vi "test_COM_comando1byte.vi"() -> ()   [LabVIEW 2019]
uses:
  <vilib>/numeric/Random Number (Range) U64.vi
  <vilib>/numeric/sub_Random U32.vi
  <vilib>/Instr/_visa.llb/VISA Configure Serial Port (Instr).vi
panel:
  out "x = y?":bool
  out "bytes enviados":u32
  out "error out":errorcluster
  out "numero de tramas\ncorrectamente recibidas":i64
  out "cmd enviado":string
  out "cmd leido":string
  in  "stop":bool
  # "ESTE VI ES PARA PROBAR LA RUTINA DE ARDUINO DE LEER \nTRAMA DE DATOS EN STANDALONE GUARDADA EN LA CARPETA:\nC:\\Trabajo_Robot\\TFG_ROBOT\\CONTROL_ROBOT\\ARDUINO_TEST_ENVIOTRAMA"
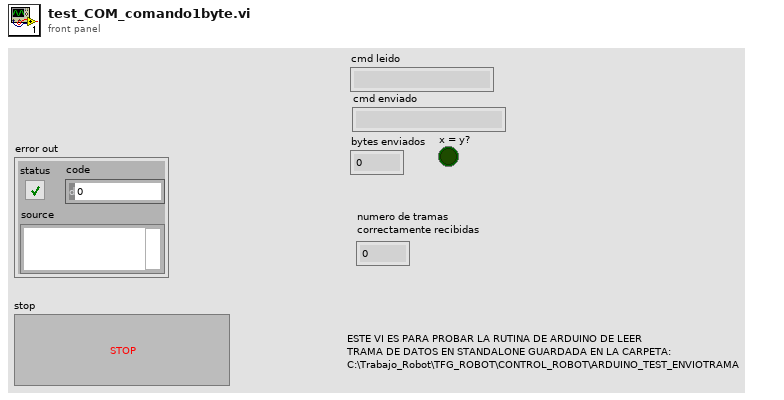
[diagram p1: front panel]
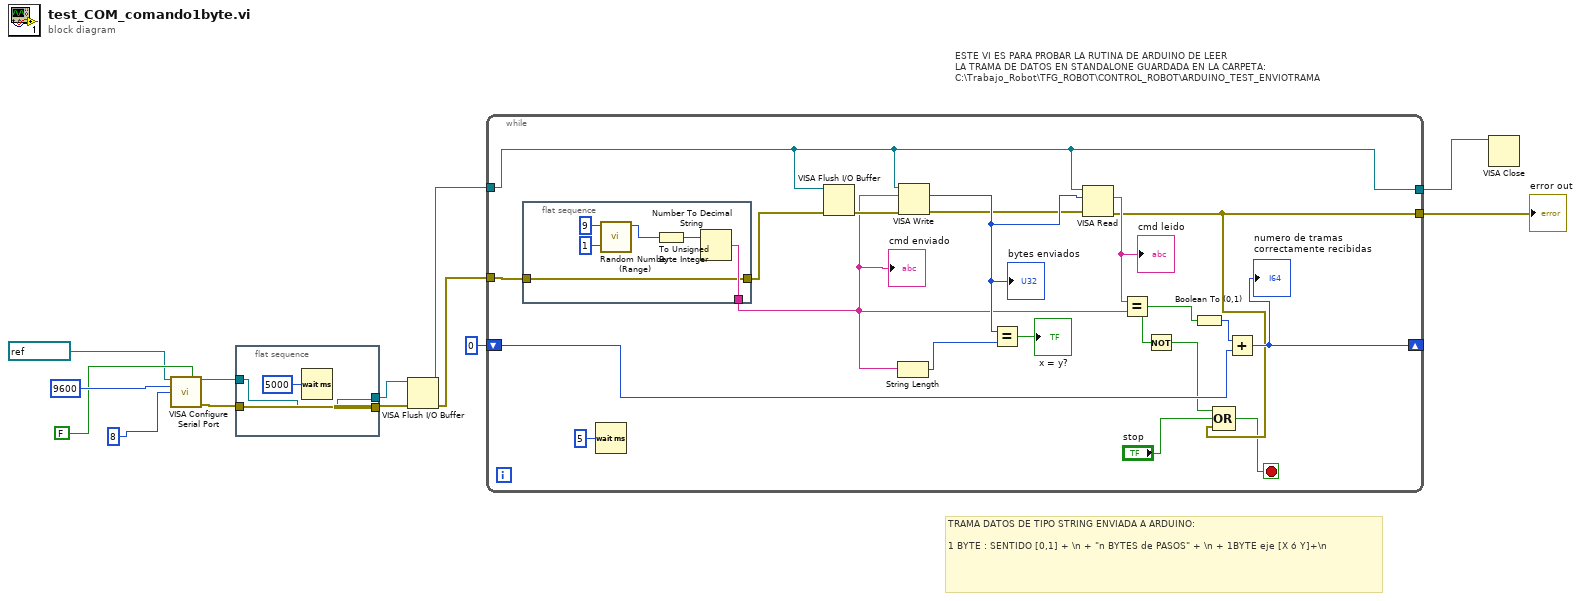
[diagram p0: block diagram]
diagram:
  # "TRAMA DATOS DE TIPO STRING ENVIADA A ARDUINO:\n\n1 BYTE : SENTIDO [0,1] + \\n + \"n BYTES de PASOS\" + \\n + 1BYTE eje [X ó Y]+\\n"
  # "ESTE VI ES PARA PROBAR LA RUTINA DE ARDUINO DE LEER \nLA TRAMA DE DATOS EN STANDALONE GUARDADA EN LA CARPETA:\nC:\\Trabajo_Robot\\TFG_ROBOT\\CONTROL_ROBOT\\ARDUINO_TEST_ENVIOTRAMA"
  n1 = call-poly "VISA Configure Serial Port"("VISA resource name"=refnum<visa-resource-name> "COM4", "Enable Termination\nChar (T)"=FALSE ("Enable Termination\nChar (T)"), "baud rate (9600)"=u32 9600, "data bits (8)"=u16 8) -> ("VISA resource name out"=w7:refnum<visa-resource-name>, "error out"=w11:errorcluster)  [unwired: 10 in]
  n2 = flat-sequence {
    tunnel: [w16] -> w8
    tunnel: w11 -> [w16]
    tunnel: [w14] -> w6
    tunnel: w7 -> [w14]
    frame #0 {
      n3 = Wait (ms)(milliseconds to wait=u32 5000) -> ()  [unwired: 1 out]
    }
  }
  n4 = VISA Flush I/O Buffer(VISA resource name=w6, error in (no error)=w8) -> (VISA resource name out=w4:refnum<visa-resource-name>, error out=w5:errorcluster)  [unwired: 1 in]
  n5 = while {
    tunnel: w5 -> [w24]
    tunnel: w4 -> [w19]
    tunnel: [w19] -> w1
    tunnel: [w26] -> w2
    shift-right: [w28] -> _
    shift-left: i16 0 -> [w29]
    stop <- w25 stop-if-true
    n6 = flat-sequence {
      tunnel: [w37] -> w17
      tunnel: w24 -> [w36]
      tunnel: [w36] -> w18
      frame #0 {
        n7 = call-poly <vilib>:"Random Number (Range).vi"("lower bound (0)"=u64 1, "upper bound (100)"=u64 9) -> ("number"=w39:u64)  [unwired: 9 in]
        n8 = To Unsigned Byte Integer(number=w39) -> (unsigned 8bit integer=w38:u8)
        n9 = Number To Decimal String(number=w38) -> (decimal integer string=w37:string)  [unwired: 1 in]
      }
    }
    n10 = Wait (ms)(milliseconds to wait=u32 5) -> ()  [unwired: 1 out]
    n11 = VISA Flush I/O Buffer(VISA resource name=w19, error in (no error)=w18) -> (error out=w35:errorcluster)  [unwired: 1 in, 1 out]
    n12 = String Length(string=w17) -> (length=w34:i32)
    n13 = VISA Write(VISA resource name=w19, write buffer=w17, error in (no error)=w35) -> (return count=w33:u32, error out=w32:errorcluster)  [unwired: 1 out]
    "bytes enviados" <- w33
    n14 = Equal?(x=w33, y=w34) -> (x = y?=→"x = y?":bool)
    n15 = VISA Read(VISA resource name=w19, byte count=w33, error in (no error)=w32) -> (read buffer=w31:string, error out=w26:errorcluster)  [unwired: 2 out]
    "cmd leido" <- w31
    n16 = Equal?(x=w31, y=w17) -> (x = y?=w21:bool)
    n17 = Not(x=w21) -> (.not. x?=w20:bool)
    n18 = Boolean To (0,1)(Boolean=w21) -> (0, 1=w30:i16)
    n19 = Compound Arithmetic op=OR(w20, "stop", w26) -> (w25:bool)
    n20 = Add(x=w30, y=w29) -> (x+y=w28:i16)
    "numero de tramas\ncorrectamente recibidas" <- w28
    "cmd enviado" <- w17
  }
  "error out" <- w2
  n21 = VISA Close(VISA resource name=w1) -> ()  [unwired: 1 in, 1 out]
